vi "Error_Helper_RaiseError.vi"(6 "Additional Info":string, 7 "Raise?":bool, 8 "Error In":errorcluster, 9 "Error To Raise":errorcluster) -> (0 "Error Out":errorcluster)   [LabVIEW 2020, in "hse-misc.lvlib"]
doc: "If <b>Raise?</b> is true, puts the error in <b>Error To Raise</b> on the error output and adds <b>Additional Info</b> to the source of the error.\n\n\n\n____\nHAMPEL SOFTWARE ENGINEERING v3.8.0 (2023-12-18 14:41)"
uses:
  hse-misc.lvlib
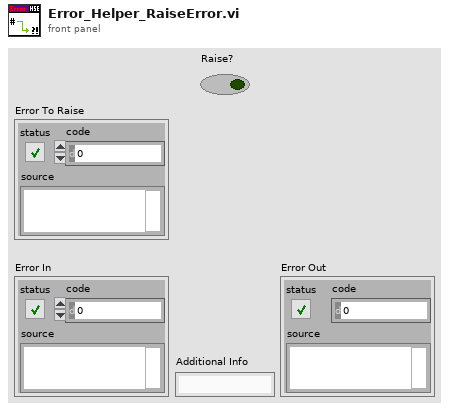
[diagram p1: front panel]
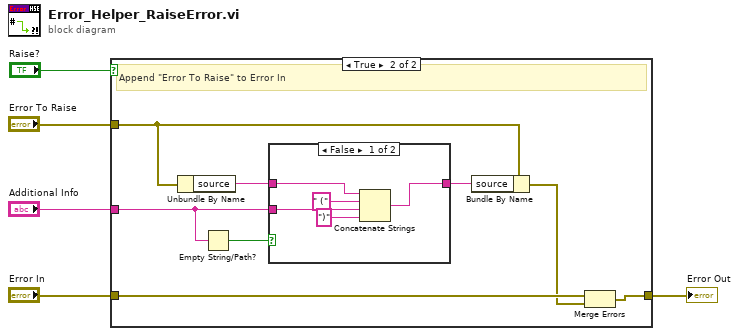
[diagram p0: block diagram]
diagram:
  n1 = case shown="True" "Raise?" {
    tunnel: [w6 w10] -> w5
    tunnel: "Additional Info" -> [_ w13]
    tunnel: "Error In" -> [w6 w12]
    tunnel: "Error To Raise" -> [_ w9]
    frame False {
      # "Do nothing"
    }
    frame True {
      # "Append \"Error To Raise\" to Error In"
      n2 = Unbundle By Name(w9) -> ("source"=w7:string)
      n3 = Empty String/Path?(string/path=w13) -> (empty?=w14:bool)
      n4 = case shown="False" w14 {
        tunnel: w13 -> [w19 _]
        tunnel: [w15 w20] -> w8
        tunnel: w7 -> [w16 w20]
        frame False {
          n5 = Concatenate Strings(w16, " (" ("string"), w19, ")" ("string")) -> (w15:string)
        }
        frame True {
        }
      }
      n6 = Bundle By Name(cluster=w9, "source"=w8) -> (w11:errorcluster)
      n7 = Merge Errors(w12, w11) -> (w10:errorcluster)
    }
  }
  "Error Out" <- w5
